vi "DoAddCoordinate.vi"(8 "error in (no error)":errorcluster, 11 "SnakeData1":T1) -> (0 "error out":errorcluster, 3 "SnakeData1 2":T1)   [LabVIEW 2019, in "RT_Game.lvlib" / "SnakeGame.lvclass"]
uses:
  SnakeGame.lvclass
  SnakeData.ctl
  Direction.ctl
  Game/Coordinate.ctl
  CoordinateData.ctl
  Game/Game.lvclass
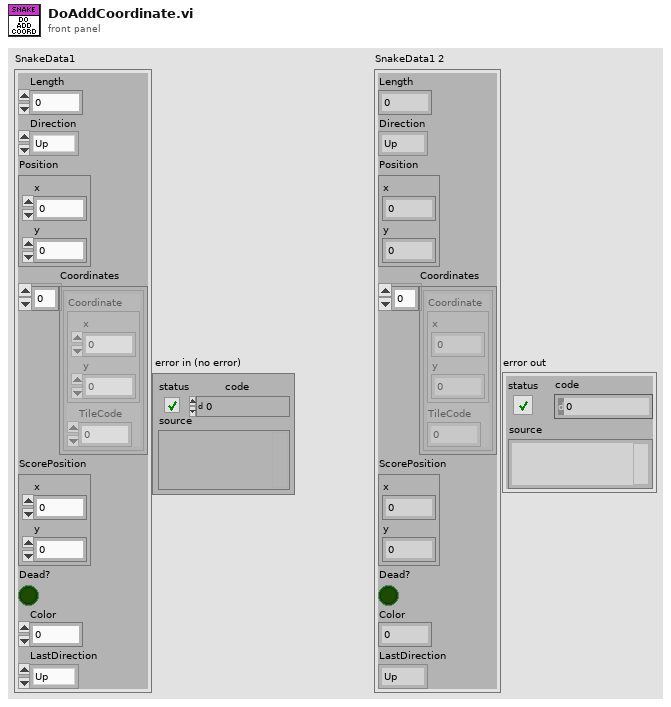
[diagram p1: front panel]
types:
  T1 = typedef "RT_Game.lvlib/SnakeGame.lvclass/SnakeData.ctl" = cluster{"Length":i16, "Direction":T2, "Position":T3, "Coordinates":T4[], "ScorePosition":T3, "Dead?":bool, "Color":fxp<+,3,3>, "LastDirection":T2}
  T2 = typedef "RT_Game.lvlib/SnakeGame.lvclass/Direction.ctl" = enum16{"Up", "Left", "Down", "Right"}
  T3 = typedef "RT_Game.lvlib/Game.lvclass/Coordinate.ctl" = cluster{"x":dbl, "y":dbl}
  T4 = typedef "RT_Game.lvlib/SnakeGame.lvclass/CoordinateData.ctl" = cluster{"Coordinate":T3, "TileCode":u16}
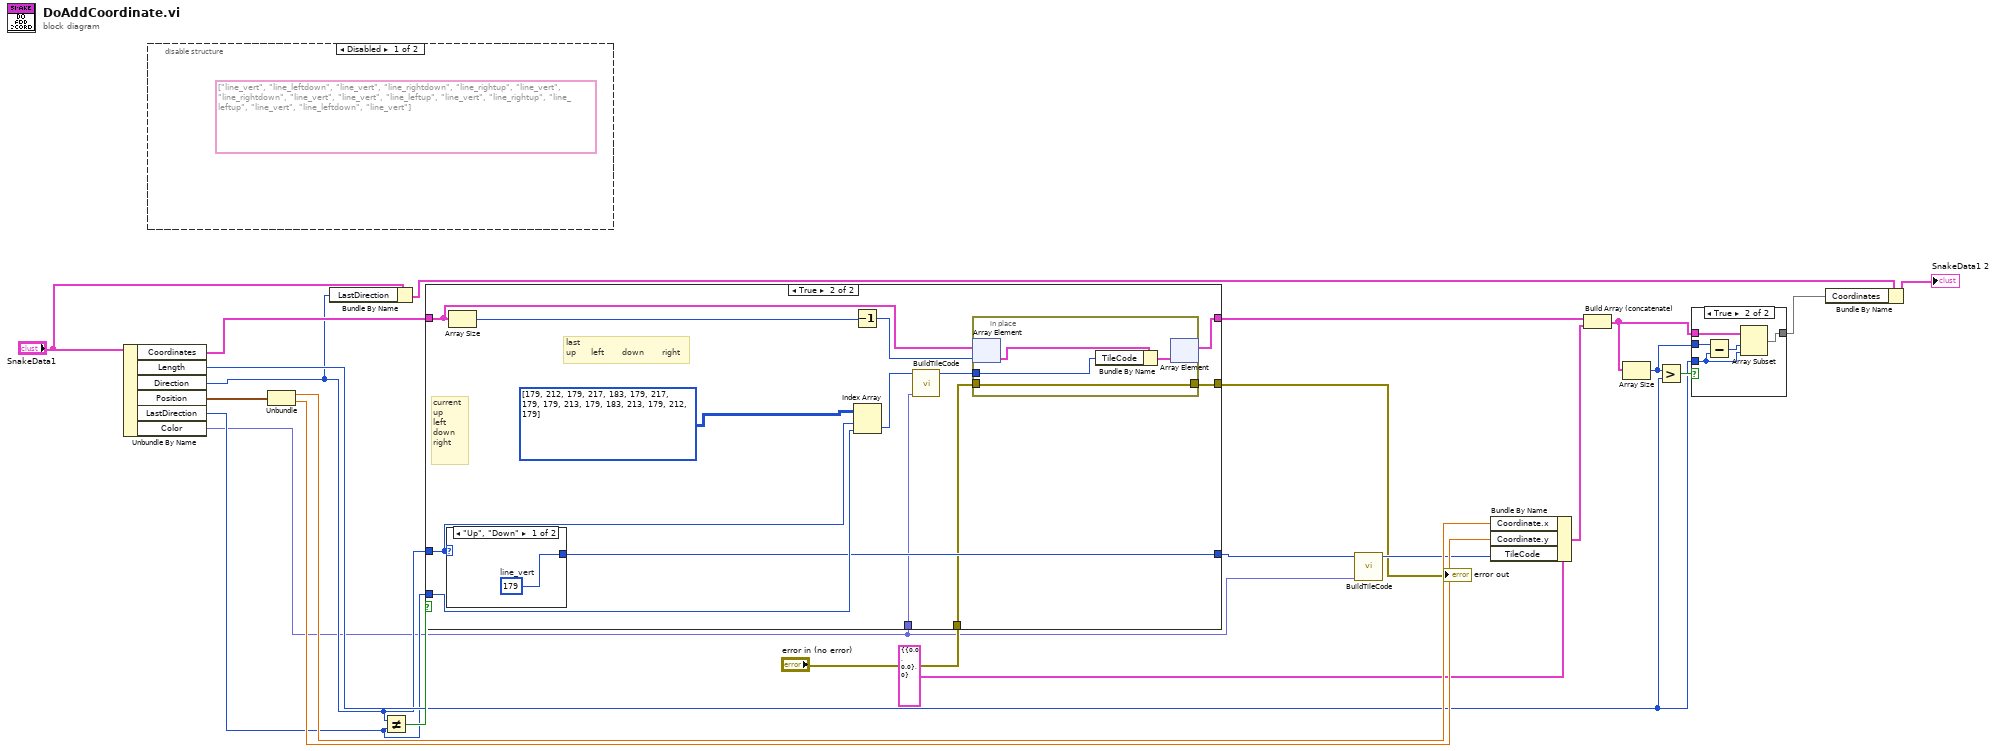
[diagram p0: block diagram]
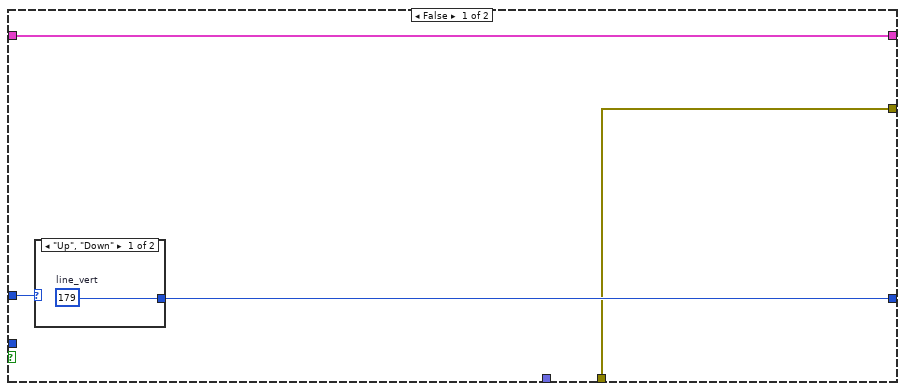
[diagram p3: hidden frame]
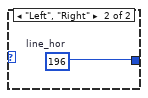
[diagram p4: hidden frame]
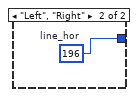
[diagram p5: hidden frame]
diagram:
  n1 = Unbundle By Name("SnakeData1") -> ("Coordinates"=w14:T4[], "Length"=w12:i16, "Direction"=w7:T2, "Position"=w13:T3, "LastDirection"=w6:T2, "Color"=w1:fxp<+,3,3>)
  n2 = disable-structure shown="Disabled" {
    frame Disabled {
      (unwired) string[][] [["line_vert", "line_leftdown", "line_vert", "line_rightdown"], ["line_rightup", "line_vert", "line_rightdown", "line_vert"], ["line_vert", "line_leftup", "line_vert", "line_rightup"], ["line_leftup", "line_vert", "line_leftdown", "line_vert"]] ("Array")
    }
    frame Enabled {
    }
  }
  n3 = Unbundle(w13) -> ("x"=w22:dbl, "y"=w23:dbl)
  n4 = Bundle By Name(cluster="SnakeData1", "LastDirection"=w7) -> (w8:T1)
  n5 = Not Equal?(x=w7, y=w6) -> (x != y?=w20:bool)
  n6 = case shown="True" w20 {
    tunnel: w7 -> [w27 w37]
    tunnel: w6 -> [_ w42]
    tunnel: [w26 w36] -> w4
    tunnel: w14 -> [w25 w39]
    tunnel: [w25 w38] -> w21
    tunnel: w1 -> [_ w31]
    tunnel: "error in (no error)" -> [w24 w33]
    tunnel: [w24 w32] -> w2
    frame False {
      n7 = case shown="\"Up\", \"Down\"" w27 {
        tunnel: [w28 w29] -> w26
        frame "Up", "Down" {
          w28 = 179  # line_vert
        }
        frame "Left", "Right" {
          w29 = u16 196  # line_hor
        }
      }
    }
    frame True {
      # "last\nup     left      down      right"
      # "current\nup\nleft\ndown\nright"
      n8 = case shown="\"Up\", \"Down\"" w37 {
        tunnel: [w43 w44] -> w36
        frame "Up", "Down" {
          w43 = 179  # line_vert
        }
        frame "Left", "Right" {
          w44 = u16 196  # line_hor
        }
      }
      n9 = Array Size(array=w39) -> (size(s)=w41:i32)
      n10 = Decrement(x=w41) -> (x-1=w40:i32)
      n11 = Index Array(array=u8[][] [[179, 212, 179, 217], [183, 179, 217, 179], [179, 213, 179, 183], [213, 179, 212, 179]] ("Array"), index (row)=w37, index (col)=w42) -> (element=w35:u8)
      n12 = call "BuildTileCode.vi"("replace_color"=w31, "tilenumber"=w35) -> ("TileCode"=w34:u16)  [unwired: 9 in]
      n13 = in-place {
        in-place-border: w34 -> [w45]
        in-place-border: w33 -> [w46]
        in-place-border: [w46] -> w32
        n14 = in-place-array #1(w39, w40) -> (w48:T4)
        n15 = Bundle By Name(cluster=w48, "TileCode"=w45) -> (w47:T4)
        n16 = in-place-array #1(w47) -> (w38:T4[])  [unwired: 1 out]
      }
    }
  }
  "error out" <- w2
  n17 = call "BuildTileCode.vi"("replace_color"=w1, "tilenumber"=w4) -> ("TileCode"=w5:u16)  [unwired: 9 in]
  n18 = Bundle By Name(cluster=T4 {"Coordinate"={"x"=0.0, "y"=0.0}, "TileCode"=0} ("Coordinate"), "Coordinate.x"=w22, "Coordinate.y"=w23, "TileCode"=w5) -> (w19:T4)
  n19 = Build Array (concatenate)(w21, w19) -> (w17:T4[])
  n20 = Array Size(array=w17) -> (size(s)=w16:i32)
  n21 = Greater?(x=w16, y=w12) -> (0:w15:bool)
  n22 = case shown="True" w15 {
    tunnel: [w49 w54] -> w9
    tunnel: w17 -> [w49 w53]
    tunnel: w16 -> [_ w52]
    tunnel: w12 -> [_ w50]
    frame False {
    }
    frame True {
      n23 = Subtract(x=w52, y=w50) -> (x-y=w51:i32)
      n24 = Array Subset(array=w53, index=w51, length=w50) -> (w54:T4[])
    }
  }
  n25 = Bundle By Name(cluster=w8, "Coordinates"=w9) -> (→"SnakeData1 2":T1)
